vi "Press Enter Key and wait.vi"(8 "error in (no error)":errorcluster, 11 "PS Driver AMI4xx in":refnum<class "PS Driver AMI4xx.lvclass">) -> (0 "error out":errorcluster, 3 "PS Driver AMI4xx out":refnum<class "PS Driver AMI4xx.lvclass">)   [LabVIEW 2020, in "PS Driver.lvlib" / "PS Driver AMI4xx.lvclass"]
uses:
  PS Driver AMI4xx.lvclass
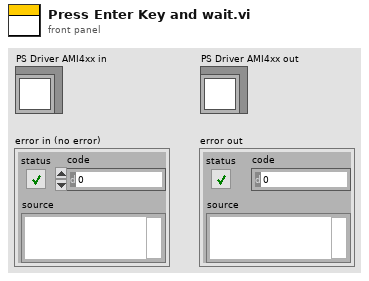
[diagram p1: front panel]
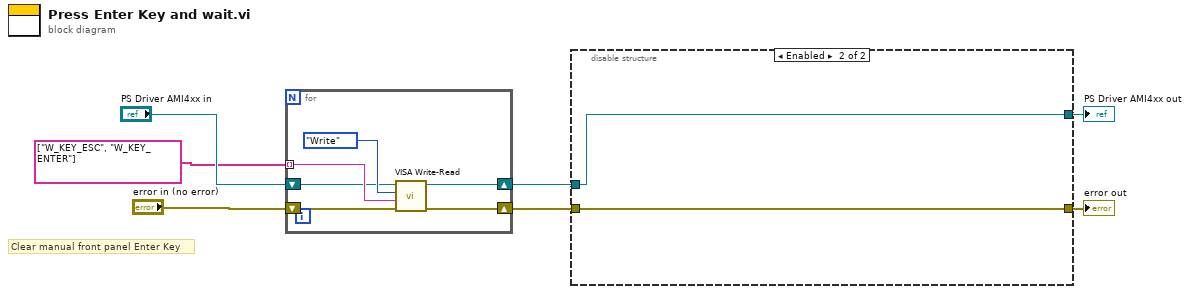
[diagram p0: block diagram]
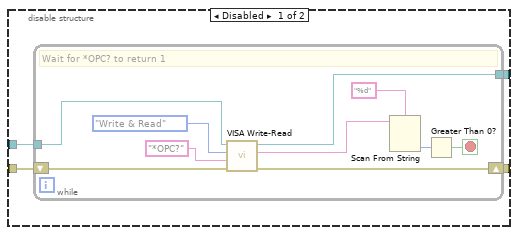
[diagram p2: hidden frame]
diagram:
  # "Clear manual front panel Enter Key"
  n1 = for {
    tunnel: string[] ["W_KEY_ESC", "W_KEY_ENTER"] -> [w13] mode=indexing
    shift-right: [w8] -> w3
    shift-left: "PS Driver AMI4xx in" -> [w11]
    shift-right: [w9] -> w4
    shift-left: "error in (no error)" -> [w10]
    n2 = call "VISA Write-Read.vi"("error in (no error)"=w10, "Command String"=w13, "Action"=enum16{"Write", "Read", "Write & Read"}."Write", "PS Driver.lvlib:PS Driver AMI4xx.lvclass"=w11) -> ("error out"=w9:errorcluster, "PS Driver.lvlib:PS Driver AMI4xx.lvclass out"=w8:refnum<class "PS Driver AMI4xx.lvclass">)  [unwired: 4 in, 2 out]
  }
  n3 = disable-structure shown="Enabled" {
    disable-tunnel: [w17 w28] -> w5
    disable-tunnel: w4 -> [w16 w28]
    disable-tunnel: w3 -> [w15 w29]
    disable-tunnel: [w14 w29] -> w2
    frame Disabled {
      n4 = while {
        shift-right: [w27] -> w17
        shift-left: w16 -> [w26]
        tunnel: w15 -> [w21]
        tunnel: [w20] -> w14
        stop <- w23 stop-if-true
        # "Wait for *OPC? to return 1"
        n5 = call "VISA Write-Read.vi"("error in (no error)"=w26, "Command String"="*OPC?", "Action"=enum16{"Write", "Read", "Write & Read"}."Write & Read", "PS Driver.lvlib:PS Driver AMI4xx.lvclass"=w21) -> ("error out"=w27:errorcluster, "Response string"=w25:string, "PS Driver.lvlib:PS Driver AMI4xx.lvclass out"=w20:refnum<class "PS Driver AMI4xx.lvclass">)  [unwired: 4 in, 1 out]
        n6 = Scan From String(format string="%d", input string=w25) -> (output 1=w22:i32)  [unwired: 3 in, 3 out]
        n7 = Greater Than 0?(x=w22) -> (x > 0?=w23:bool)
      }
    }
    frame Enabled {
    }
  }
  "PS Driver AMI4xx out" <- w2
  "error out" <- w5
